vi "Phase - Remove Frequency Offset.vi"(0 "Phase In":cluster{"t0":dbl, "dt":dbl, "Y":dbl[]}={"t0"=0.0, "dt"=1.0, "Y"=[]} {"Y" min=0.0 max=127.0 format="%.2f"; "dt" format="%.2f"; "t0" format="%.2f"}, 11 "Error In":errorcluster) -> (4 "Phase Out":cluster{"t0":dbl, "dt":dbl, "Y":dbl[]}={"t0"=0.0, "dt"=1.0, "Y"=[]} {"Y" min=0.0 max=127.0 format="%.6f"; "dt" format="%.2f"; "t0" format="%.2f"}, 15 "Error Out":errorcluster)   [LabVIEW 2019]
uses:
  <vilib>/Analysis/NI_AALPro.lvlib
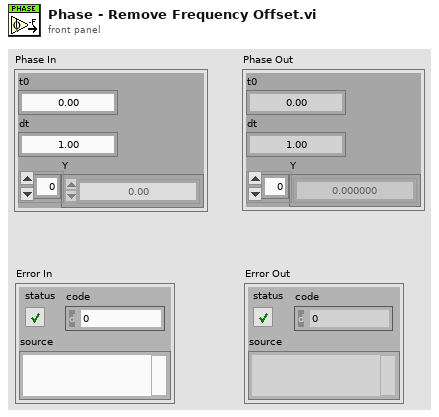
[diagram p1: front panel]
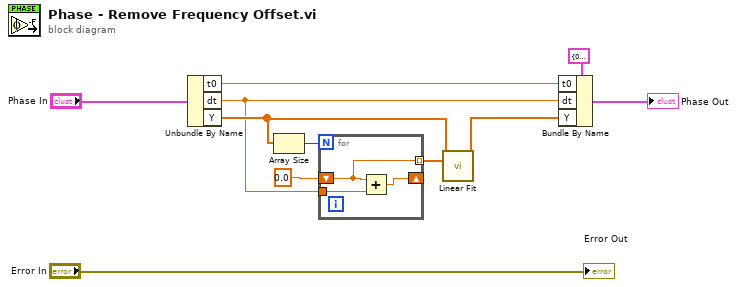
[diagram p0: block diagram]
diagram:
  n1 = Unbundle By Name("Phase In") -> ("t0"=w9:dbl, "dt"=w2:dbl, "Y"=w3:dbl[])
  n2 = Array Size(array=w3) -> (size(s)=w6:i32)
  n3 = for {
    N: w6 -> [_]
    shift-right: [w14] -> _
    shift-left: 0.0 -> [w13]
    tunnel: [w13] -> w5 mode=indexing
    tunnel: w2 -> [w12]
    n4 = Add(x=w13, y=w12) -> (x+y=w14:dbl)
  }
  n5 = call <vilib>:"Linear Fit.vi"("Y"=w3, "X"=w5) -> ("Best Linear Fit"=w1:dbl[])  [unwired: 9 in, 4 out]
  n6 = Bundle By Name(cluster=cluster{"t0":dbl, "dt":dbl, "Y":dbl[]} {"t0"=0.0, "dt"=1.0, "Y"=[]} ("Magnitude Out"), "t0"=w9, "dt"=w2, "Y"=w1) -> (→"Phase Out":cluster{"t0":dbl, "dt":dbl, "Y":dbl[]})
  "Error Out" <- "Error In"
